vi "Configure Spectrometer Channel.vi"(7 "Enable Channel Rotation (F:Disable)":bool, 8 "error in (no error)":errorcluster, 10 "Channel Number (0:Channel 0)":u16(ring) items=["Channel 0", "Channel 1", "Channel 2", "Channel 3", "Channel 4", "Channel 5", "Channel 6", "Channel 7"], 11 "VISA resource name":refnum<visa-resource-name>) -> (0 "error out":errorcluster, 3 "VISA resource name out":refnum<visa-resource-name>)   [LabVIEW 2012, in "Ocean Optics 2000 4000.lvlib"]
doc: "Sets the ADC1000-USB Spectrometer channel to the desired S2000 Unit\n\n<B> Note: </B>\n- If the rotation feature is enabled, the pixel resolution is reduced by the number of channels rotated through"
uses:
  Ocean Optics 2000 4000.lvlib
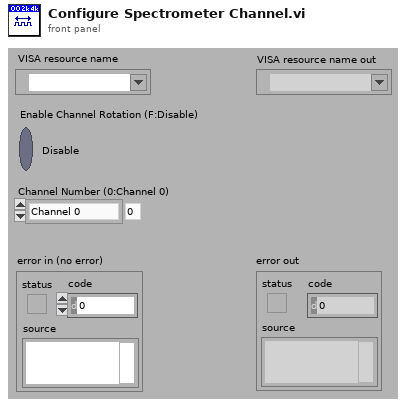
[diagram p1: front panel]
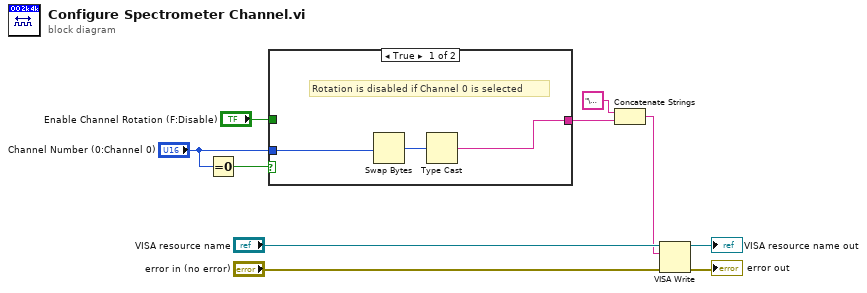
[diagram p0: block diagram]
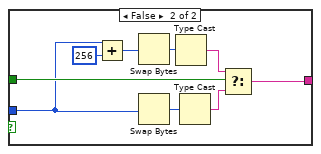
[diagram p2: hidden frame]
diagram:
  n1 = Equal To 0?(x="Channel Number (0:Channel 0)") -> (x = 0?=w4:bool)
  n2 = case shown="True" w4 {
    tunnel: "Enable Channel Rotation (F:Disable)" -> [_ w16]
    tunnel: "Channel Number (0:Channel 0)" -> [w13 w15]
    tunnel: [w11 w14] -> w2
    frame True {
      # "Rotation is disabled if Channel 0 is selected"
      n3 = Swap Bytes(anything=w13) -> (byte swapped=w12:u16)
      n4 = Type Cast(x=w12) -> (*(type *) &x=w11:string)  [unwired: 1 out]
    }
    frame False {
      n5 = Add(x=w15, y=u16 256) -> (x+y=w18:u16)
      n6 = Swap Bytes(anything=w18) -> (byte swapped=w17:u16)
      n7 = Swap Bytes(anything=w15) -> (byte swapped=w19:u16)
      n8 = Type Cast(x=w17) -> (*(type *) &x=w21:string)  [unwired: 1 out]
      n9 = Type Cast(x=w19) -> (*(type *) &x=w20:string)  [unwired: 1 out]
      n10 = Select(t=w21, s=w16, f=w20) -> (s? t:f=w14:string)
    }
  }
  n11 = Concatenate Strings("\u000b", w2) -> (w1:string)
  n12 = VISA Write(VISA resource name="VISA resource name", write buffer=w1, error in (no error)="error in (no error)") -> (VISA resource name out=→"VISA resource name out":refnum<visa-resource-name>, error out=→"error out":errorcluster)  [unwired: 1 out]
